vi "parsing test program.vi"() -> ()   [LabVIEW 2020]
uses:
  <vilib>/regexp/Match Regular Expression.xnode
panel:
  out "submatch 3":string
  out "submatch 2":string
  out "submatch 1":string
  in  "input string":string
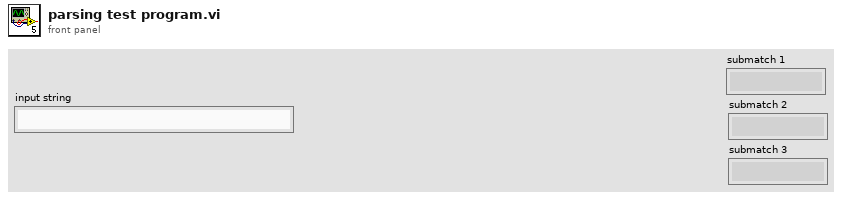
[diagram p1: front panel]
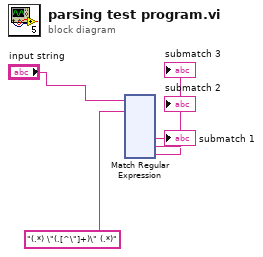
[diagram p0: block diagram]
diagram:
  n1 = xnode "Match Regular Expression"("input string"="input string", "regular expression"="(.*) \"(.[^\"]+)\" (.*)") -> ("submatch 1"=→"submatch 1":string, "submatch 2"=→"submatch 2":string, "submatch 3"=→"submatch 3":string)  [unwired: 4 in, 5 out]
